vi "TreeNode Get NumChildren.vi"(8 "error in (no error)":errorcluster, 11 "TreeNode DVR in":refnum<data-value>) -> (0 "error out":errorcluster, 2 "NumChildren":i32, 3 "TreeNode DVR out":refnum<data-value>)   [LabVIEW 2012, in "MDSplus.lvlib"]
uses:
  <vilib>/MDSplus/Classes/Data_Class/TreeNode_Class/TreeNode.lvclass
  <vilib>/MDSplus/Library/MDSplus.lvlib
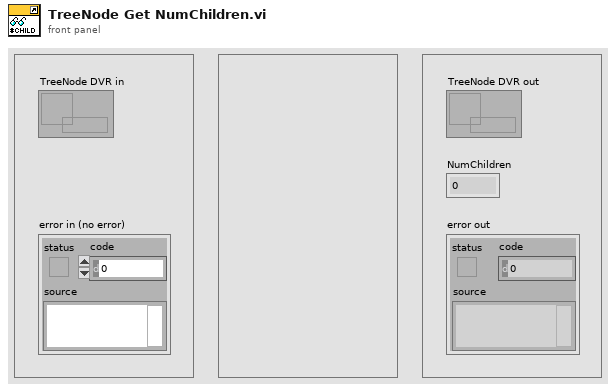
[diagram p1: front panel]
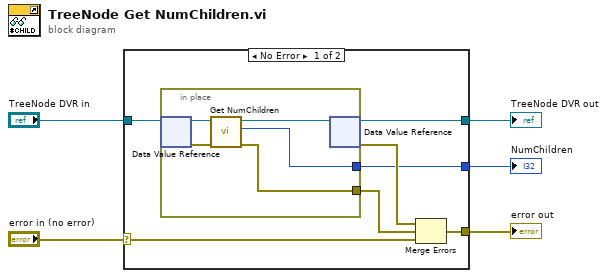
[diagram p0: block diagram]
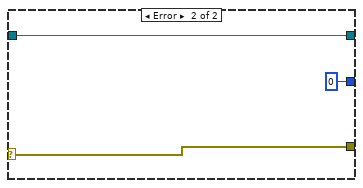
[diagram p2: hidden frame]
diagram:
  n1 = case shown="No Error" "error in (no error)" {
    selector: "error in (no error)" -> [w11 w20]
    tunnel: "TreeNode DVR in" -> [w12 w19]
    tunnel: [w8 w20] -> w5
    tunnel: [w9 w19] -> w2
    tunnel: [w6 0 ("NID")] -> w1
    frame No Error {
      n2 = in-place {
        in-place-border: [w15] -> w7
        in-place-border: [w13] -> w6
        n3 = in-place-dvr #1(w12) -> (w17:refnum<class "TreeNode.lvclass">, w16:errorcluster)
        n4 = call-dynamic "Get NumChildren.vi"("error in (no error)"=w16, "TreeNode in"=w17) -> ("error out"=w15:errorcluster, "NumChildren"=w13:i32, "TreeNode out"=w14:refnum<class "TreeNode.lvclass">)  [unwired: 7 in]
        n5 = in-place-dvr #1(w14) -> (w9:refnum<data-value>, w10:errorcluster)
      }
      n6 = Merge Errors(w10, w7, w11) -> (w8:errorcluster)
    }
    frame Error {
    }
  }
  "error out" <- w5
  "TreeNode DVR out" <- w2
  "NumChildren" <- w1
